vi "Get Actual Malleable VI Name.vi"(8 "error in":errorcluster, 11 "VI Reference":refnum<vi>) -> (0 "error out":errorcluster, 3 "Malleable VI Full Qualified Name":string)   [LabVIEW 2020, in "Peek Window.lvlib" / "Malleable VI Type.lvclass"]
uses:
  VI Types/Malleable VI Type/Malleable VI Type.lvclass
  8898ce48-ddb9-4dd9-ab7b-7e2c6aebdd87.vi
  VI Types/Malleable VI Type/Malleable VI Type.lvclass/Malleable VI Type.ctl
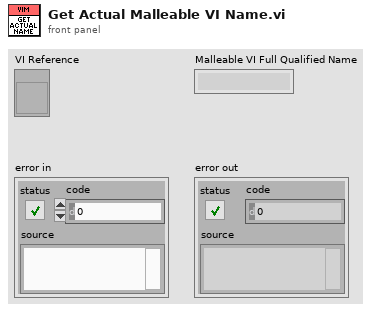
[diagram p1: front panel]
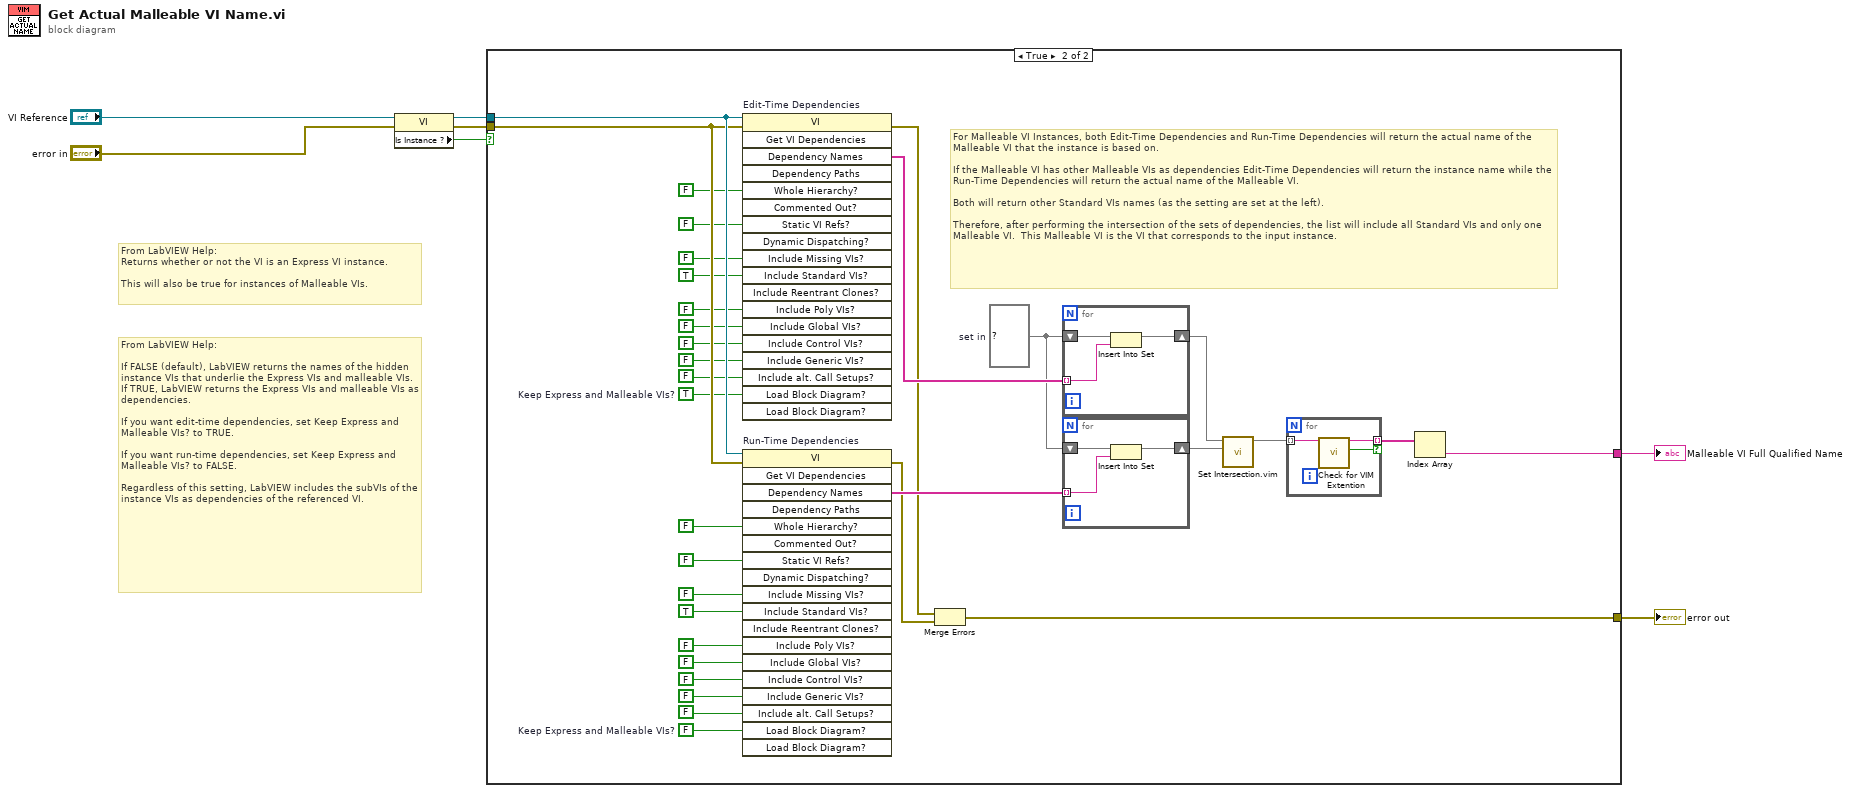
[diagram p0: block diagram]
diagram:
  # "From LabVIEW Help:\nReturns whether or not the VI is an Express VI instance.\n\nThis will also be true for instances of Malleable VIs."
  # "From LabVIEW Help:\n\nIf FALSE (default), LabVIEW returns the names of the hidden instance VIs that underlie the Express VIs and malleable VIs. If TRUE, LabVIEW returns the Express VIs and malleable VIs as dependencies.\n\nIf you want edit-time dependencies, set Keep Express and Malleable VIs? to TRUE. \n\nIf you want run-time dependencies, set Keep Express and Malleable VIs? to FALSE. \n\nRegardless of this setting, LabVIEW includes the subVIs of the instance VIs as dependencies of the referenced VI."
  n1 = property class="VI"(reference="VI Reference", error in="error in") -> (reference out=w7:refnum<vi>, error out=w5:errorcluster, "Is Instance ?"=w1:bool)
  n2 = case shown="True" w1 {
    tunnel: w7 -> [_ w41]
    tunnel: [_ w40] -> w6
    tunnel: w5 -> [w8 w39]
    tunnel: [w8 w38] -> w4
    frame False {
    }
    frame True {
      w13 = set{string} {}  # set in
      w18 = FALSE  # Keep Express and Malleable VIs?
      w37 = TRUE  # Keep Express and Malleable VIs?
      # "For Malleable VI Instances, both Edit-Time Dependencies and Run-Time Dependencies will return the actual name of the Malleable VI that the instance is based on.  \n\nIf the Malleable VI has other Malleable VIs as dependencies Edit-Time Dependencies will return the instance name while the Run-Time Dependencies will return the actual name of the Malleable VI.\n\nBoth will return other Standard VIs names (as the setting are set at the left).\n\nTherefore, after performing the intersection of the sets of dependencies, the list will include all Standard VIs and only one Malleable VI.  This Malleable VI is the VI that corresponds to the input instance."
      n3 = invoke on="Edit-Time Dependencies" class="VI" method="Get VI Dependencies"(reference=w41, error in=w39, "Whole Hierarchy?"=FALSE, "Static VI Refs?"=FALSE, "Include Missing VIs?"=FALSE, "Include Standard VIs?"=TRUE, "Include Poly VIs?"=FALSE, "Include Global VIs?"=FALSE, "Include Control VIs?"=FALSE, "Include Generic VIs?"=FALSE, "Include alt. Call Setups?"=FALSE, "Load Block Diagram?"=w37) -> (error out=w10:errorcluster, "Dependency Names"=w17:string[])  [unwired: 7 in, 17 out]
      n4 = invoke on="Run-Time Dependencies" class="VI" method="Get VI Dependencies"(reference=w41, error in=w39, "Whole Hierarchy?"=FALSE, "Static VI Refs?"=FALSE, "Include Missing VIs?"=FALSE, "Include Standard VIs?"=TRUE, "Include Poly VIs?"=FALSE, "Include Global VIs?"=FALSE, "Include Control VIs?"=FALSE, "Include Generic VIs?"=FALSE, "Include alt. Call Setups?"=FALSE, "Load Block Diagram?"=w18) -> (error out=w9:errorcluster, "Dependency Names"=w12:string[])  [unwired: 7 in, 17 out]
      n5 = Merge Errors(w10, w9) -> (w38:errorcluster)
      n6 = for {
        shift-right: [w44] -> w16
        shift-left: w13 -> [w43]
        tunnel: w17 -> [w42] mode=indexing
        n7 = Insert Into Set(10:w42, 11:w43) -> (3:w44:set{string})  [unwired: 1 out]
      }
      n8 = for {
        shift-right: [w47] -> w11
        shift-left: w13 -> [w46]
        tunnel: w12 -> [w45] mode=indexing
        n9 = Insert Into Set(10:w45, 11:w46) -> (3:w47:set{string})  [unwired: 1 out]
      }
      n10 = call "Set Intersection.vim"("set 2"=w11, "set 1"=w16) -> ("intersection"=w15:set{string})  [unwired: 9 in]
      n11 = for {
        tunnel: w15 -> [w48] mode=indexing
        tunnel: [w49] -> w14 mode=indexing if=w50
        n12 = call "Check for VIM Extention.vi"("VI Name in"=w48) -> ("Is a Malleable VI"=w50:bool, "VI Name out"=w49:string)  [unwired: 9 in]
      }
      n13 = Index Array(array=w14) -> (element=w40:string)  [unwired: 1 in]
    }
  }
  "error out" <- w4
  "Malleable VI Full Qualified Name" <- w6
